vi "modifyRow.vi"(0 "reference in":refnum<class "Project Panels.lvclass">, 2 "Row In":string[](array[string]), 5 "error in (no error)":errorcluster) -> (14 "reference out":refnum<class "Project Panels.lvclass">, 16 "Row":string[](array[string]), 17 "Cancel?":bool, 19 "error out":errorcluster)   [LabVIEW 2015, in "Project Panels.lvclass"]
uses:
  Project Panels.lvclass
panel:
  in  "Cancel Button":bool
  in  "Quantity:":string
  in  "Description:":string
  in  "S/N:":string
  in  "P/N:":string
  in  "OK Button":bool
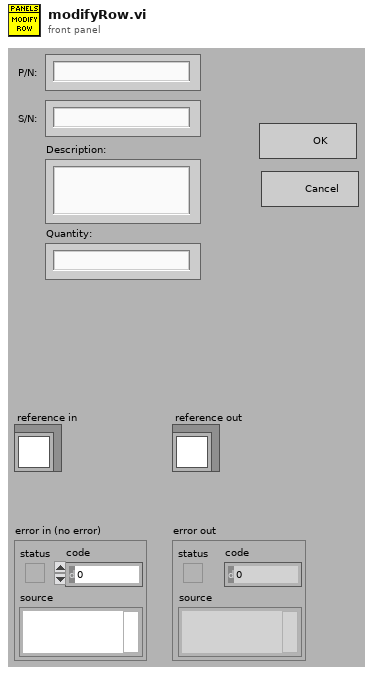
[diagram p1: front panel]
types:
  T1 = typedef "Project Panels.lvclass/ObjectAttributesRef.ctl" = refnum<data-value>
  T2 = typedef "Project Panels.lvclass/ObjectAttributes.ctl" = cluster{"MyAttribute":dbl, "device_controller_ref":refnum<class "Devices Controller.lvclass">, "file_controller_ref":refnum<class "File Controller.lvclass">, "item_controller_ref":refnum<class "Items Controller.lvclass">, "item_tables":cluster{"checkIN":string[][], "checkOUT":string[][], "storage":string[][]}, "quickbook_table":cluster{"notes":string[][]}, "notification_controller_ref":refnum<class "Notification Controller.lvclass">, "partstracking_controller_ref":refnum<class "PartsTracking Controller.lvclass">, "product_tables":cluster{"k4b2":string[][], "fitmate":string[][], "RMR":string[][], "CPET":string[][], "BP":string[][], "PP":string[][], "k5":string[][], "bb-pft":string[][]}, "rowsColour":u32[], "low_resolution?":bool, "run_python?":bool}
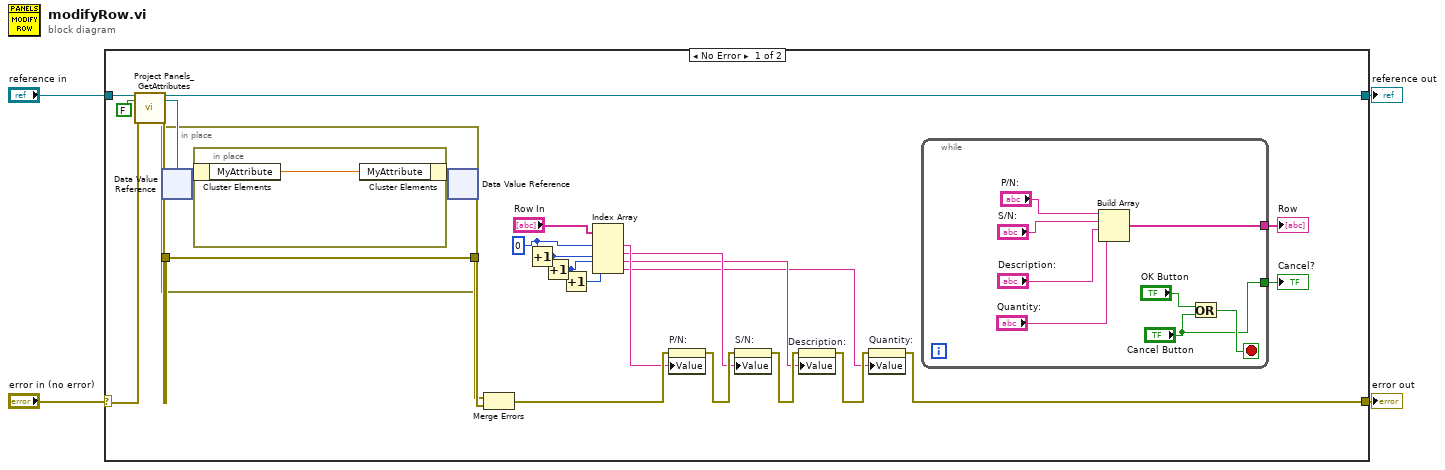
[diagram p0: block diagram]
diagram:
  n1 = case shown="No Error" "error in (no error)" {
    selector: "error in (no error)" -> [w24 w42]
    tunnel: [w11 w42] -> w3
    tunnel: [w22 w41] -> w1
    tunnel: "reference in" -> [w26 w41]
    frame No Error {
      w18 = 0 ("index")
      n2 = call "Project Panels_GetAttributes.vi"("reference in"=w26, "return data? (T)"=FALSE, "error in (no error)"=w24) -> ("reference out"=w22:refnum<class "Project Panels.lvclass">, "attributes ref"=w21:T1, "error out"=w23:errorcluster)  [unwired: 13 in, 1 out]
      n3 = in-place {
        in-place-border: w23 -> [w37]
        in-place-border: [w37] -> w27
        n4 = in-place-dvr #1(w21) -> (w38:T2)  [unwired: 1 out]
        n5 = in-place {
          n6 = in-place-cluster #2(w38) -> ("MyAttribute"=w40:dbl)
          n7 = in-place-cluster #2("MyAttribute"=w40) -> (w39:T2)
        }
        n8 = in-place-dvr #1(w39) -> (w28:errorcluster)  [unwired: 1 out]
      }
      n9 = Merge Errors(w27, w28) -> (w14:errorcluster)
      n10 = Increment(x=w18) -> (x+1=w17:i32)
      n11 = Increment(x=w17) -> (x+1=w15:i32)
      n12 = Increment(x=w15) -> (x+1=w16:i32)
      n13 = Index Array(array="Row In", index #1=w18, index #2=w17, index #3=w15, index #4=w16) -> (element #1=w13:string, element #2=w7:string, element #3=w6:string, element #4=w5:string)
      n14 = property on="P/N:" class="Str"(error in=w14, "Value"=w13) -> (error out=w9:errorcluster)  [unwired: 1 in, 1 out]
      n15 = property on="S/N:" class="Str"(error in=w9, "Value"=w7) -> (error out=w8:errorcluster)  [unwired: 1 in, 1 out]
      n16 = property on="Description:" class="Str"(error in=w8, "Value"=w6) -> (error out=w10:errorcluster)  [unwired: 1 in, 1 out]
      n17 = property on="Quantity:" class="Str"(error in=w10, "Value"=w5) -> (error out=w11:errorcluster)  [unwired: 1 in, 1 out]
      n18 = while {
        tunnel: [w32] -> w20
        tunnel: ["Cancel Button"] -> w12
        stop <- w30 stop-if-true
        n19 = Build Array("P/N:", "S/N:", "Description:", "Quantity:") -> (w32:string[])
        n20 = Or(x="OK Button", y="Cancel Button") -> (x .or. y?=w30:bool)
      }
      "Row" <- w20
      "Cancel?" <- w12
    }
    frame Error {
    }
  }
  "error out" <- w3
  "reference out" <- w1
